vi "frame de minu (1).vi"() -> ()   [LabVIEW 2021]
uses:
  <vilib>/Instr/_visa.llb/VISA Configure Serial Port (Instr).vi
panel:
  in  "stop":bool
  out "Tank":dbl(slide) scale=0.0..300.0
  out "String 2":string
  in  "VISA resource name":refnum<visa-resource-name>
  in  "REFRESH":bool
  # "EQUIPO ROSA MACHO MECATRÓNIXXX"
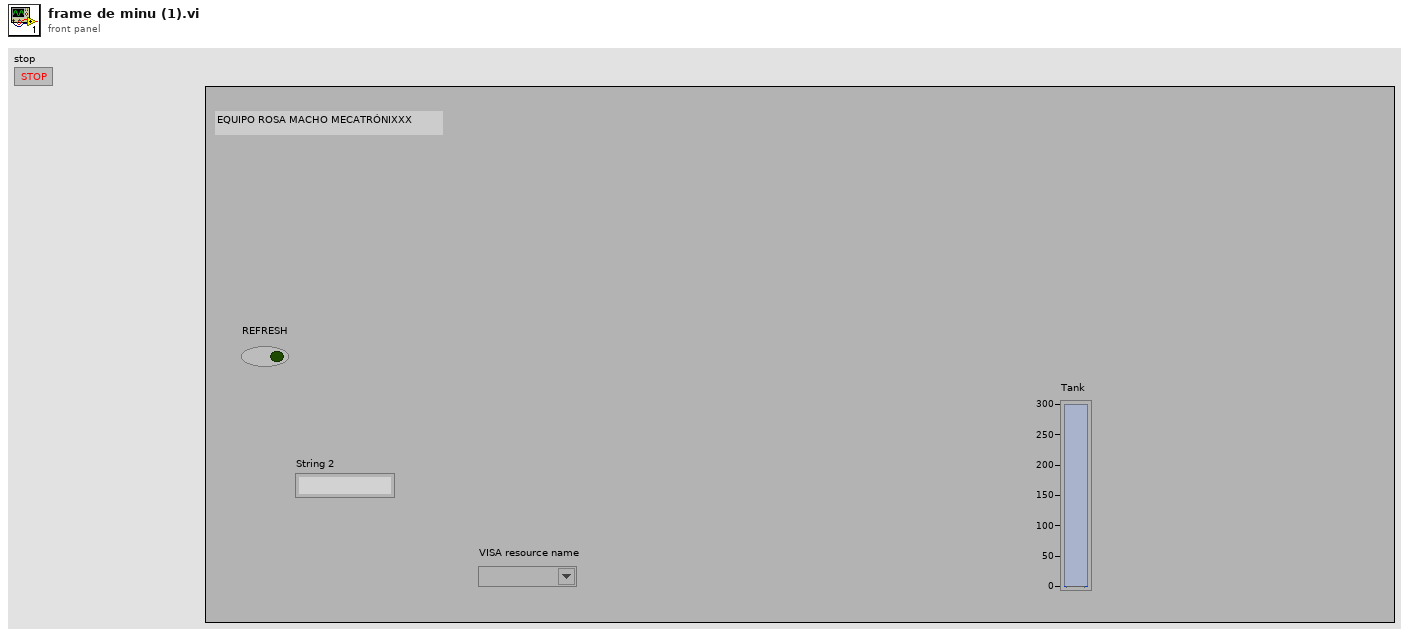
[diagram p1: front panel]
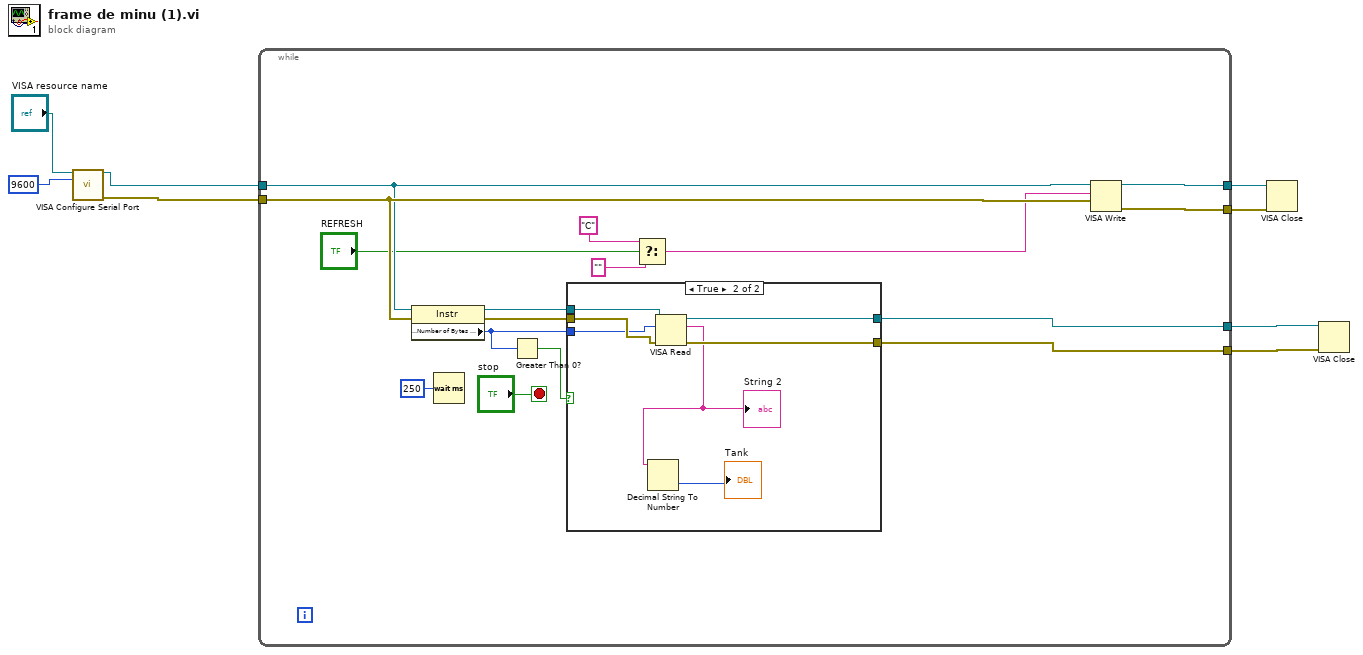
[diagram p0: block diagram]
diagram:
  n1 = call-poly "VISA Configure Serial Port"("VISA resource name"="VISA resource name", "baud rate (9600)"=u32 9600) -> ("VISA resource name out"=w8:refnum<visa-resource-name>, "error out"=w6:errorcluster)  [unwired: 12 in]
  n2 = while {
    tunnel: w8 -> [w15]
    tunnel: [w24] -> w7
    tunnel: w6 -> [w16]
    tunnel: [w23] -> w5
    tunnel: [w21] -> w2
    tunnel: [w20] -> w1
    stop <- "stop" stop-if-true
    n3 = property class="Instr"(reference=w15, error in=w16) -> (reference out=w19:refnum<visa-resource-name>, error out=w14:errorcluster, "Serial Settings:Number of Bytes at Serial Port"=w10:u32)
    n4 = Wait (ms)(milliseconds to wait=u32 250) -> ()  [unwired: 1 out]
    n5 = Greater Than 0?(x=w10) -> (x > 0?=w11:bool)
    n6 = case shown="True" w11 {
      tunnel: [w26 w33] -> w21
      tunnel: [w25 w32] -> w20
      tunnel: w19 -> [w26 w31]
      tunnel: w14 -> [w25 w30]
      tunnel: w10 -> [_ w28]
      frame False {
      }
      frame True {
        n7 = VISA Read(VISA resource name=w31, byte count=w28, error in (no error)=w30) -> (VISA resource name out=w33:refnum<visa-resource-name>, read buffer=w29:string, error out=w32:errorcluster)  [unwired: 1 out]
        "String 2" <- w29
        n8 = Decimal String To Number(string=w29) -> (number=→"Tank":i32)  [unwired: 2 in, 1 out]
      }
    }
    n9 = Select(t="C", s="REFRESH", f="") -> (s? t:f=w13:string)
    n10 = VISA Write(VISA resource name=w15, write buffer=w13, error in (no error)=w16) -> (VISA resource name out=w24:refnum<visa-resource-name>, error out=w23:errorcluster)  [unwired: 1 out]
  }
  n11 = VISA Close(VISA resource name=w7, error in (no error)=w5) -> ()  [unwired: 1 out]
  n12 = VISA Close(VISA resource name=w2, error in (no error)=w1) -> ()  [unwired: 1 out]
